vi "Convert Version String to Cluster.vi"(11 "Version":string) -> (2 "Version Valid?":bool, 3 "Version":cluster{i32, i32, i32})   [LabVIEW 2025, in "Protection and Counter Addon Shared.lvlib"]
uses:
  Protection and Counter Addon Shared.lvlib
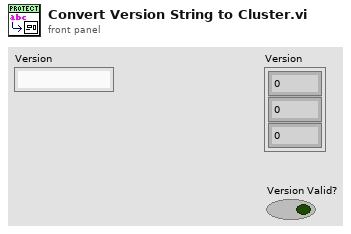
[diagram p1: front panel]
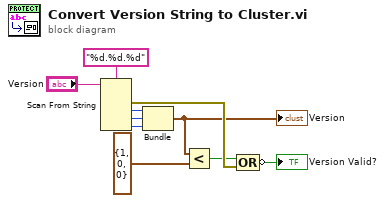
[diagram p0: block diagram]
diagram:
  n1 = Scan From String(format string="%d.%d.%d", input string="Version") -> (error out=w9:errorcluster, output 1=w3:i32, output 2=w4:i32, output 3=w1:i32)  [unwired: 5 in, 2 out]
  n2 = Bundle(w3, w4, w1) -> (w6:cluster{i32, i32, i32})  [unwired: 1 in]
  "Version" <- w6
  n3 = Less?(x=w6, y=cluster{i32, i32, i32} {1, 0, 0} ("output cluster")) -> (x < y?=w8:bool)
  n4 = Compound Arithmetic op=OR(w8, w9) -> (invert →"Version Valid?":bool)
